vi "_io_query_long_data.vi"(4 "Simulation read buffer (\"Simulation\")":string="Simulation", 6 "Block Logging (F)":bool, 7 "Trim Response End":bool=TRUE, 8 "error in":errorcluster caption="error in (no error)", 9 "Max chunk read bytes count (65536)":u32=65536, 10 "Write buffer":string, 11 "VISA resource name":refnum<visa-resource-name>) -> (0 "error out":errorcluster, 2 "Read buffer":string, 3 "VISA resource name out":refnum<visa-resource-name>)   [LabVIEW 2020, in "Rohde&Schwarz RTx Oscilloscopes.lvlib" / "rsidr_core.lvlib"]
uses:
  rsidr_core.lvlib
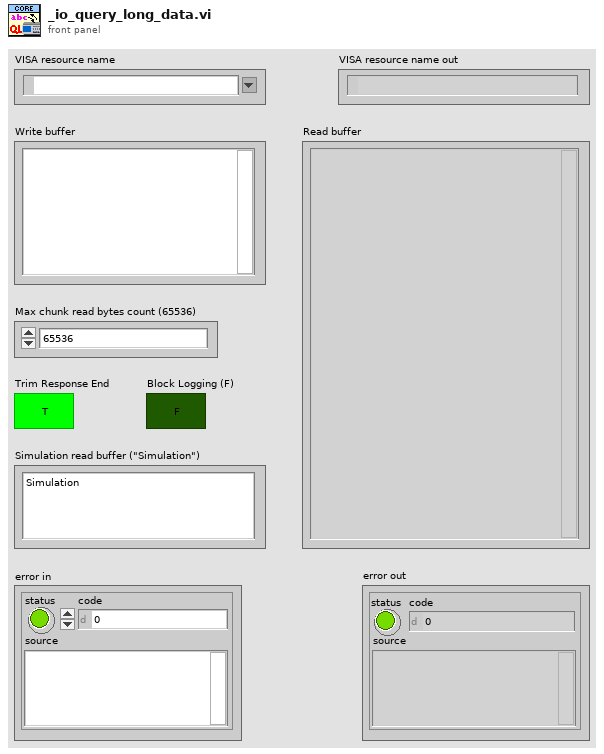
[diagram p1: front panel]
types:
  T1 = typedef "Rohde&Schwarz RTx Oscilloscopes.lvlib/rsidr_core.lvlib/type_Session_Data.ctl" = cluster{"IDN string":string, "Instrument FW":string, "Instr type":string, "Instr type for err. msg.":string, "Installed Options":string[], "Ignore Error Messages":string, "Logging params":variant, "OPC Timeout":i32, "VISA Timeout":i32, "STB Poll VISA Timeout":i32, "Additional Flags":i32, "Wait Before Read":i32, "Wait Before Write":i32, "Option String Flags":i32, "IO Segment Size":i64, "VISA Access Mode":T2, "Interface Type":T3, "OPC Wait Mode":T4, "Bin Float Number  Format":T5, "Bin Integer Number Format":T6, "Simulate":bool, "VXIcapable":bool, "Duplicate Session":bool, "Add LF to Write":bool, "Logging":bool, "Fast Sweep":bool, "Query Instrument Status":bool, "Check Range":bool, "Check Options":bool, "OPC-sync Attr Writes":bool, "OPC-sync Attr Queries":bool}
  T2 = typedef "Rohde&Schwarz RTx Oscilloscopes.lvlib/rsidr_core.lvlib/type_VisaAccessMode.ctl" = u16
  T3 = typedef "Rohde&Schwarz RTx Oscilloscopes.lvlib/rsidr_core.lvlib/type_InterfaceType.ctl" = enum16{"Unknown", "GPIB", "VXI", "GPIB_VXI", "ASRL", "PXI", "TCPIP", "USB", "SOCKET"}
  T4 = typedef "Rohde&Schwarz RTx Oscilloscopes.lvlib/rsidr_core.lvlib/type_OPC_Wait_Mode.ctl" = enum16{"STBpolling", "STBpollingSlow", "STBpollingSuperSlow", "ServiceRequest", "OPCquery"}
  T5 = typedef "Rohde&Schwarz RTx Oscilloscopes.lvlib/rsidr_core.lvlib/type_Binary_Float_Number_Format.ctl" = enum16{"Float_4_Bytes_Swapped", "Float_4_Bytes", "Double_8_Bytes_Swapped", "Double_8_Bytes"}
  T6 = typedef "Rohde&Schwarz RTx Oscilloscopes.lvlib/rsidr_core.lvlib/type_Binary_Integer_Number_Format.ctl" = enum16{"Int32_4_Bytes_Swapped", "Int32_4 Bytes", "Int16_2_Bytes_Swapped", "Int16_2_Bytes"}
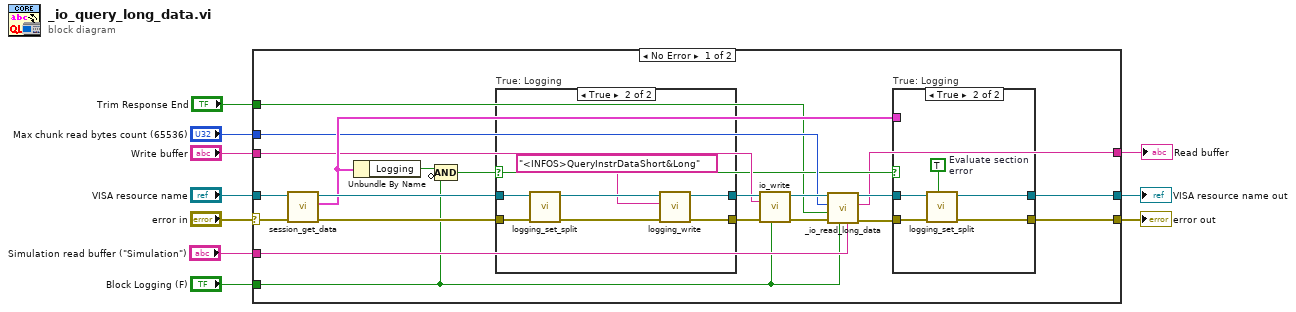
[diagram p0: block diagram]
diagram:
  n1 = case shown="No Error" "error in" {
    selector: "error in" -> [w21 w49]
    tunnel: [w16 w48] -> w4
    tunnel: [w17 w49] -> w3
    tunnel: "Write buffer" -> [w19 _]
    tunnel: "VISA resource name" -> [w22 w48]
    tunnel: "Max chunk read bytes count (65536)" -> [w18 _]
    tunnel: "Simulation read buffer (\"Simulation\")" -> [w20 _]
    tunnel: [w12 _] -> w5
    tunnel: "Block Logging (F)" -> [w14 _]
    tunnel: "Trim Response End" -> [w11 _]
    frame No Error {
      n2 = call "session_get_data.vi"("error in"=w21, "VISA resource name"=w22) -> ("error out"=w27:errorcluster, "Session User Data out"=w23:T1, "VISA resource name out"=w26:refnum<visa-resource-name>)  [unwired: 6 in, 1 out]
      n3 = Unbundle By Name(w23) -> ("Logging"=w13:bool)
      n4 = Compound Arithmetic op=AND(w13, invert w14) -> (w15:bool)
      n5 = case "True: Logging" shown="True" w15 {
        tunnel: w27 -> [w40 w45]
        tunnel: w26 -> [w39 w44]
        tunnel: [w40 w47] -> w28
        tunnel: [w39 w46] -> w29
        frame False {
        }
        frame True {
          n6 = call "logging_set_split.vi"("error in"=w45, "VISA resource name"=w44) -> ("error out"=w43:errorcluster, "VISA resource name out"=w42:refnum<visa-resource-name>)  [unwired: 8 in]
          n7 = call "logging_write.vi"("error in"=w43, "String to write"="<INFOS>QueryInstrDataShort&Long" ("format string"), "VISA resource name"=w42) -> ("error out"=w47:errorcluster, "VISA resource name out"=w46:refnum<visa-resource-name>)  [unwired: 7 in]
        }
      }
      n8 = call "io_write.vi"("Block Logging (F)"=w14, "error in"=w28, "write buffer"=w19, "VISA resource name"=w29) -> ("error out"=w30:errorcluster, "VISA resource name out"=w31:refnum<visa-resource-name>)  [unwired: 6 in]
      n9 = call "_io_read_long_data.vi"("Simulation read buffer (\"Simulation\")"=w20, "Block Logging (F)"=w14, "error in"=w30, "Trim Response End (T)"=w11, "Max segment read bytes count (65536)"=w18, "VISA resource name"=w31) -> ("error out"=w25:errorcluster, "Read buffer"=w12:string, "VISA resource name out"=w24:refnum<visa-resource-name>)  [unwired: 2 in, 1 out]
      n10 = case "True: Logging" shown="True" w15 {
        tunnel: w25 -> [w33 w38]
        tunnel: [w33 w36] -> w17
        tunnel: w24 -> [w32 w37]
        tunnel: [w32 w35] -> w16
        tunnel: w23 -> [_ _]
        frame False {
        }
        frame True {
          w34 = TRUE  # Evaluate section error
          n11 = call "logging_set_split.vi"("Evaluate section error (F)"=w34, "error in"=w38, "VISA resource name"=w37) -> ("error out"=w36:errorcluster, "VISA resource name out"=w35:refnum<visa-resource-name>)  [unwired: 7 in]
        }
      }
    }
    frame Error {
    }
  }
  "VISA resource name out" <- w4
  "error out" <- w3
  "Read buffer" <- w5
